vi "FGV_Kommunikation.vi"(8 "error in":errorcluster, 9 "termination char\n(0xA = '\\n' = LF)  2":u8=3 caption="Endzeichen\n(0xA = '\\n' = LF)" format="%.0x", 10 "Aktion":T1, 11 "VISA":refnum<visa-resource-name> caption="VISA-Ressourcenname") -> (0 "error out":errorcluster, 1 "Gase":cluster{string, i32}[][](array[cluster]), 3 "Device":string, 4 "Array 2":string[][][](array[string]), 5 "Array 3":string[][](array[string]))   [LabVIEW 2020, in "Linearisierung v2.lvlib" / "Gasteiler.lvlib" / "HovaCal.lvlib"]
uses:
  HovaCal.lvlib
  Aktion_FGV_Kom.ctl
  Aktion_txt.ctl
  Aktion_FGV_Betriebsdaten.ctl
  Betriebsdaten.ctl
  Vaporizer.ctl
  Dynamsiche_Werte.ctl
  <vilib>/Instr/_visa.llb/VISA Configure Serial Port (Instr).vi
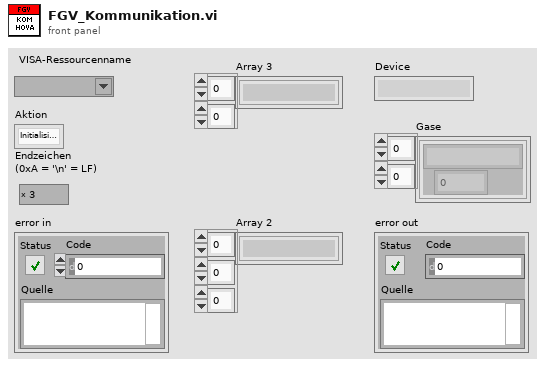
[diagram p1: front panel]
types:
  T1 = typedef "Linearisierung v2.lvlib/Gasteiler.lvlib/HovaCal.lvlib/Aktion_FGV_Kom.ctl" = enum16{"Initialisieren", "Betriebsparameter", "Gase", "Vaporizer", "Dynamische Werte", "Beenden", "Com ändern", "Gase init"}
  T2 = typedef "Linearisierung v2.lvlib/Gasteiler.lvlib/HovaCal.lvlib/Aktion_txt.ctl" = enum16{"ini", "lesen"}
  T3 = typedef "Linearisierung v2.lvlib/Gasteiler.lvlib/HovaCal.lvlib/Betriebsdaten.ctl" = cluster{"Gesamtdurchfluss":dbl, "Eingangskonzentration \nTrägergas":dbl, "Eingangskonzentration\nKomponente 1":dbl, "Eingangskonzentration \nKomponente 2":dbl, "Ausgangskonzentration \nKomponente 1 ":dbl, "Ausgangskonzentration\nKomponente 2":dbl, "l/min -> ml/min":bool, "N2 %->ppm":bool, "Komp1 ppm->%":bool, "Komp2ppm->%":bool, "Sollkomp1ppm->%":bool, "Sollkomp2ppm->%":bool}
  T4 = typedef "Linearisierung v2.lvlib/Gasteiler.lvlib/HovaCal.lvlib/Aktion_FGV_Betriebsdaten.ctl" = enum16{"Lesen", "Sollwerte schreiben", "Sollwerte lesen", "Gase schreiben", "Gase lesen", "Dynamische Werte", "GaseRef", "Gase aendern"}
  T5 = enum16{"Lesen", "Vaporizer lesen", "Vaporizer schreiben"}
  T6 = typedef "Linearisierung v2.lvlib/Gasteiler.lvlib/HovaCal.lvlib/Vaporizer.ctl" = cluster{"Pumpe Ein/Aus":dbl, "Wasser / Reagent":dbl, "Reagent dry / wet":dbl, "Reagent":dbl, "min. Temperatur\n160 °C":dbl, "Solltemperatur":dbl, "Wasserkonzentration\nSoll":dbl}
  T7 = typedef "Linearisierung v2.lvlib/Gasteiler.lvlib/HovaCal.lvlib/Dynamsiche_Werte.ctl" = cluster{"Durchfluss":dbl, "Drehzahl":dbl, "Wasserkonz.":dbl, "Ist - Temp":dbl, "Ist Konz 1":dbl, "Ist Konz 2":dbl}
  T8 = cluster{"Gesamtdurchfluss":bool, "Eingangskonzentration \nTrägergas":bool, "Eingangskonzentration\nKomponente 1":bool, "Eingangskonzentration \nKomponente 2":bool, "Ausgangskonzentration \nKomponente 1 ":bool, "Ausgangskonzentration\nKomponente 2":bool, "l/min -> ml/min":bool, "N2 %->ppm":bool, "Komp1 ppm->%":bool, "Komp2ppm->%":bool, "Sollkomp1ppm->%":bool, "Sollkomp2ppm->%":bool}
  T9 = typedef "Linearisierung v2.lvlib/Gasteiler.lvlib/HovaCal.lvlib/Gase.ctl" = cluster{"Trägergas":u16, "Komponente 1":u16, "Komponente 2":u16}
  T10 = cluster{"Pumpe Ein/Aus":bool, "Wasser / Reagent":bool, "Reagent dry / wet":bool, "Reagent":bool, "min. Temperatur\n160 °C":bool, "Solltemperatur":bool, "Wasserkonzentration\nSoll":bool}
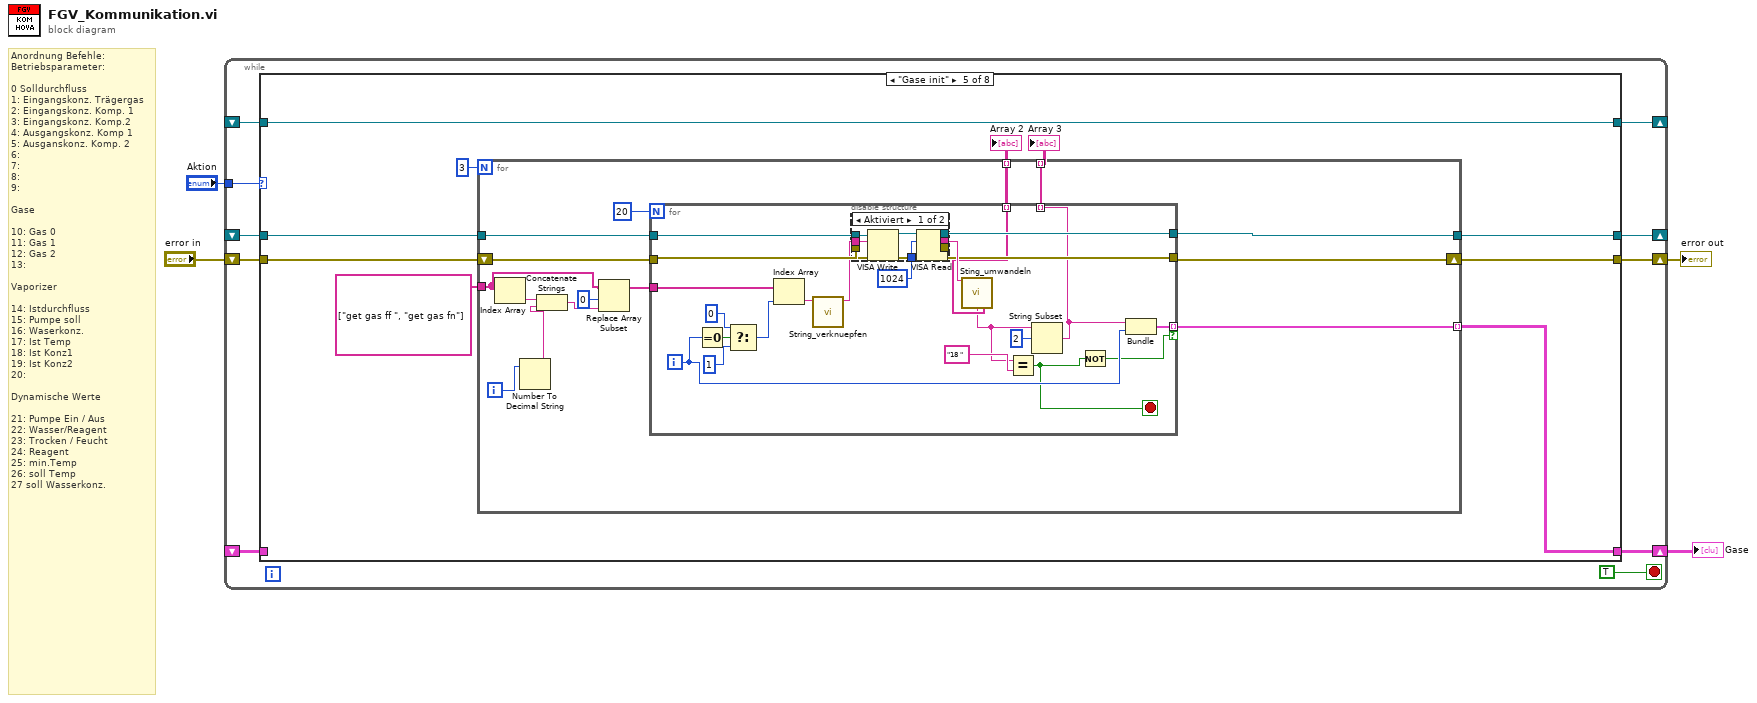
[diagram p0: block diagram]
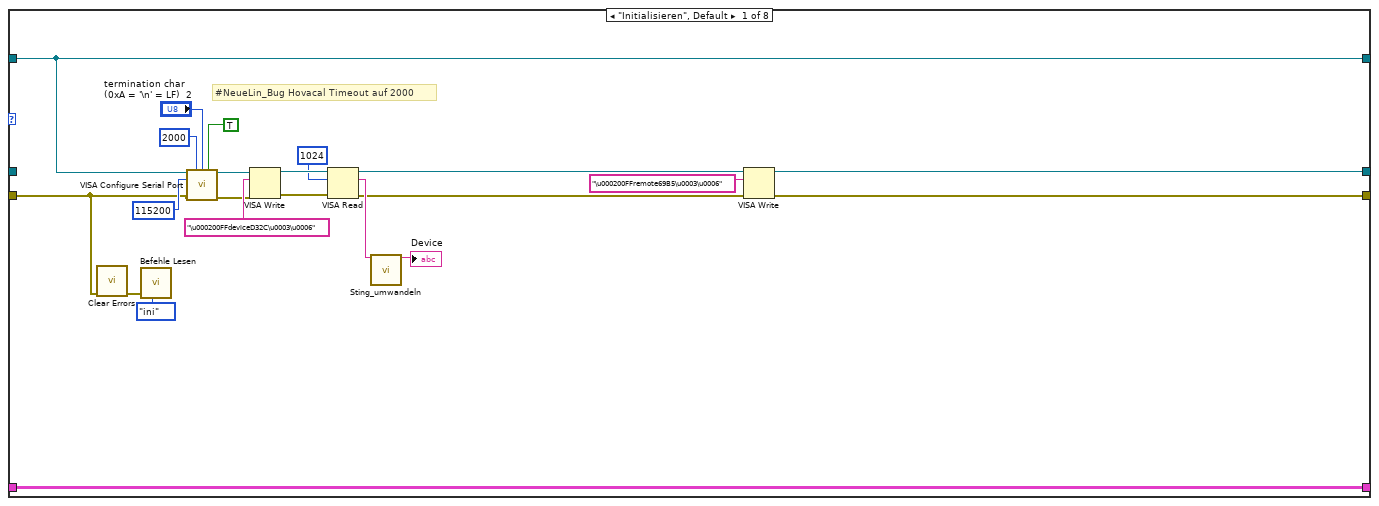
[diagram p2: hidden frame]
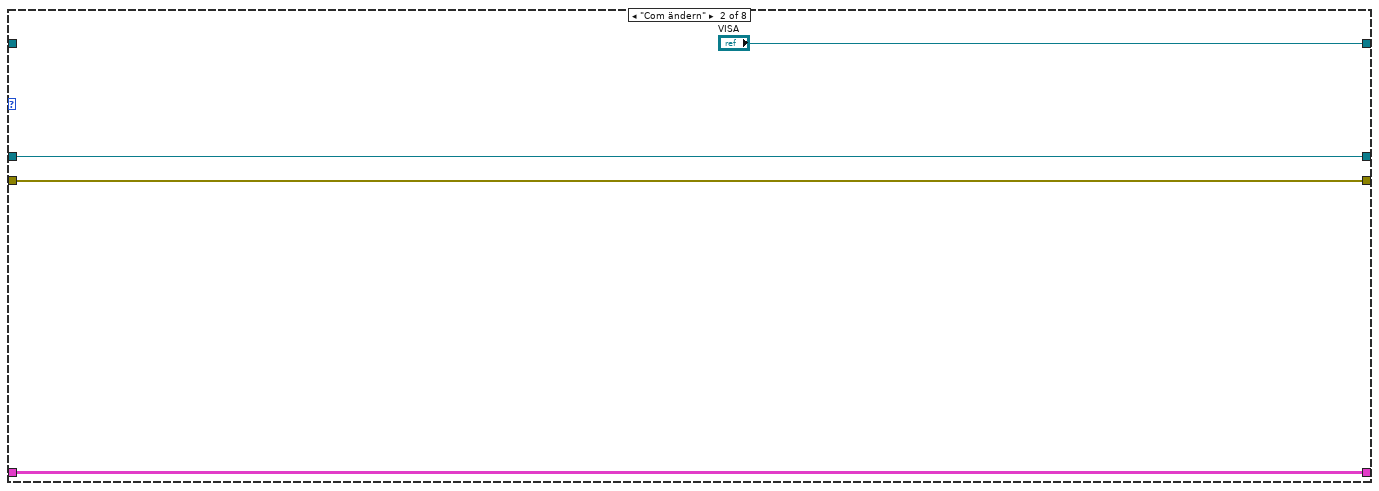
[diagram p3: hidden frame]
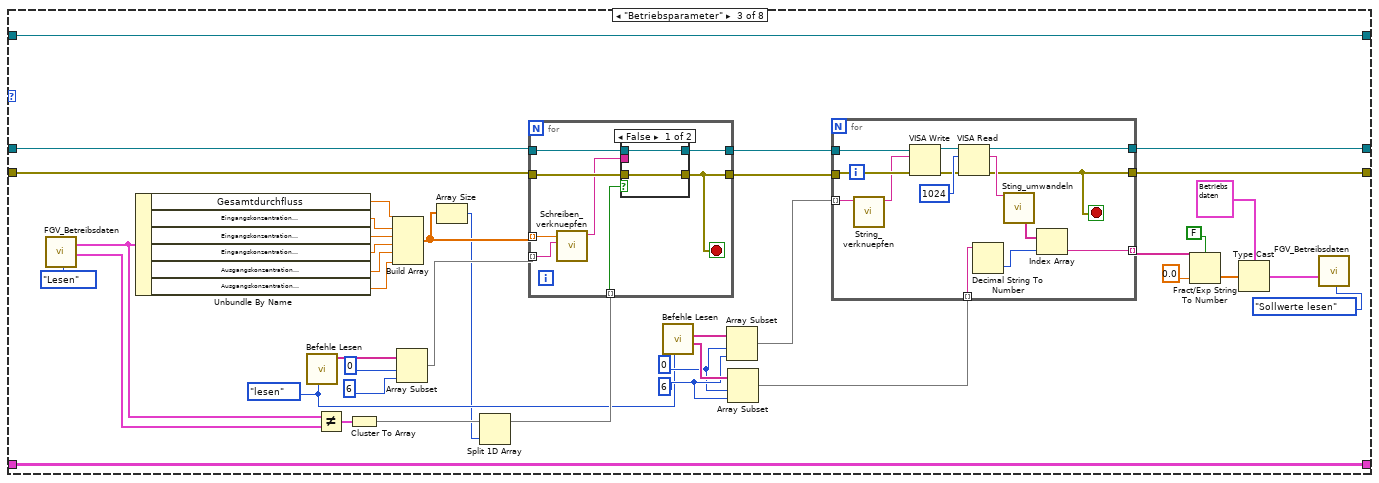
[diagram p4: hidden frame]
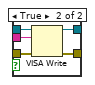
[diagram p5: hidden frame]
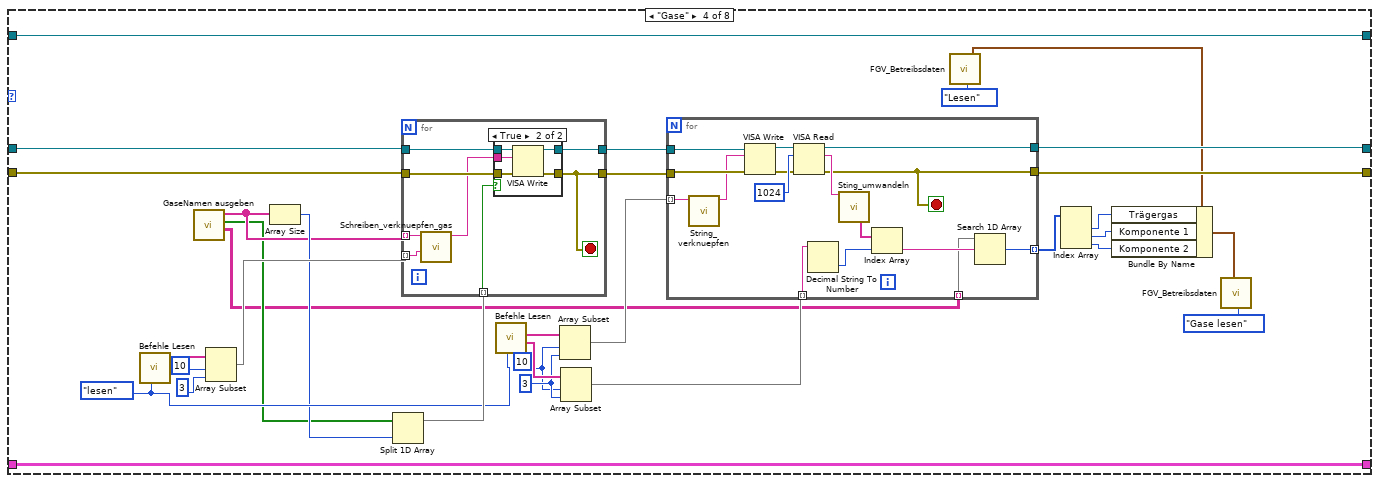
[diagram p6: hidden frame]
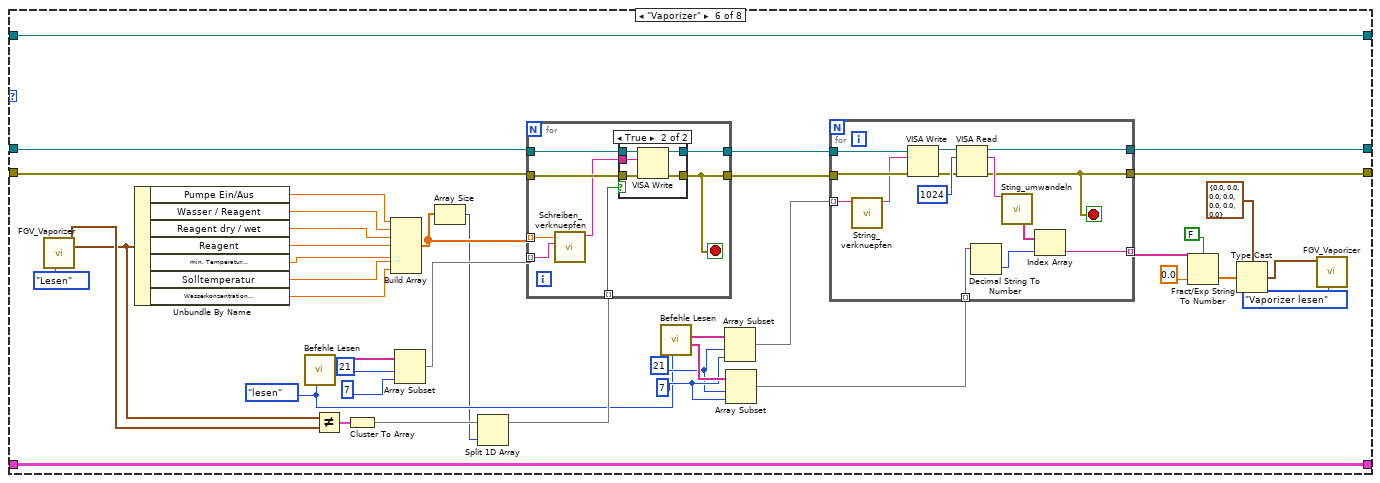
[diagram p9: hidden frame]
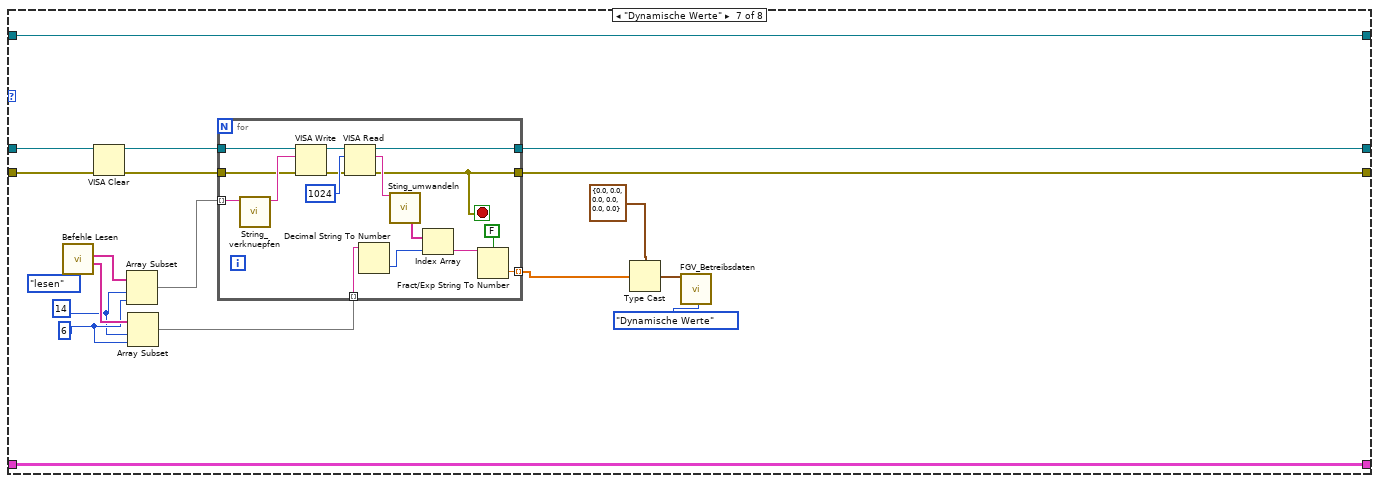
[diagram p11: hidden frame]
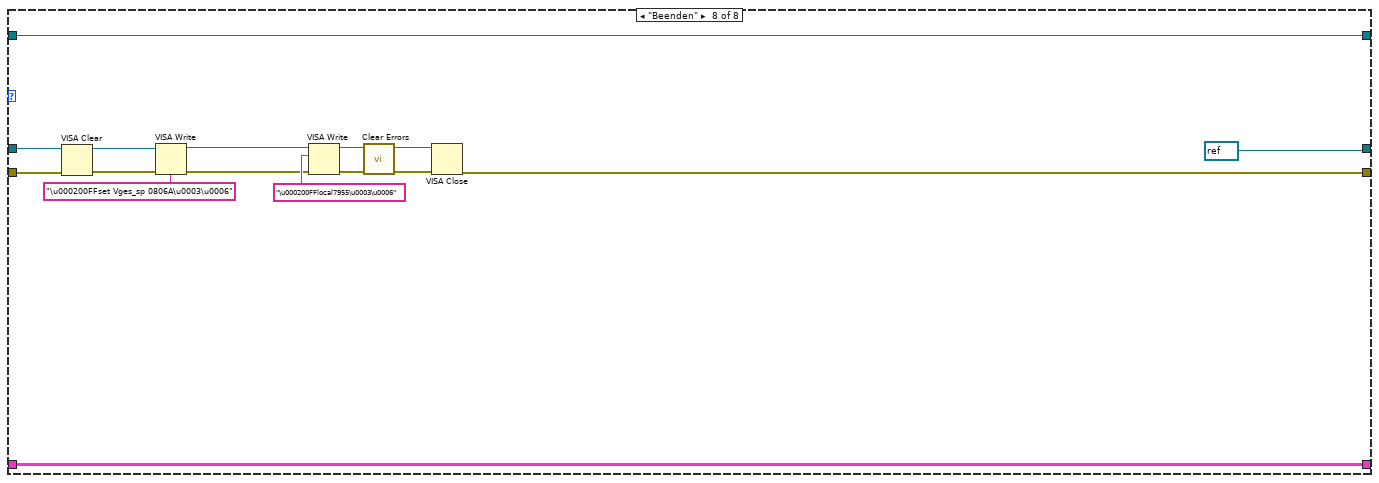
[diagram p12: hidden frame]
diagram:
  # "Anordnung Befehle:\nBetriebsparameter:\n\n0 Solldurchfluss\n1: Eingangskonz. Trägergas\n2: Eingangskonz. Komp. 1\n3: Eingangskonz. Komp.2\n4: Ausgangskonz. Komp 1\n5: Ausganskonz. Komp. 2\n6:\n7:\n8:\n9:\n\nGase\n\n10: Gas 0\n11: Gas 1\n12: Gas 2\n13:\n\nVaporizer\n\n14: Istdurchfluss\n15: Pumpe soll\n16: Waserkonz.\n17: Ist Temp\n18: Ist Konz1\n19: Ist Konz2\n20:\n\nDynamische Werte\n\n21: Pumpe Ein / Aus\n22: Wasser/Reagent\n23: Trocken / Feucht\n24: Reagent\n25: min.Temp\n26: soll Temp\n27 soll Wasserkonz."
  n1 = while {
    shift-right: [w13] -> _
    shift-left: _ -> [w11]
    shift-right: [w12] -> w4
    shift-left: "error in" -> [w10]
    tunnel: "Aktion" -> [w9]
    shift-right: [w8] -> _
    shift-left: _ -> [w7]
    shift-right: [w6] -> w1
    shift-left: _ -> [w5]
    stop <- TRUE stop-if-true
    n2 = case shown="\"Gase init\"" w9 {
      tunnel: [w24 w38 w69 w126 w180 w244 w308 refnum<visa-resource-name> refnum ("VISA resource name out")] -> w13
      tunnel: [w23 w40 w68 w125 w179 w243 w307 w336] -> w12
      tunnel: w11 -> [_ w38 w74 w128 w182 w246 w309 w340]
      tunnel: w10 -> [w15 w40 w75 w127 w181 w245 w304 w337]
      tunnel: [w18 "VISA" w44 w122 w178 w230 w302 w335] -> w8
      tunnel: w7 -> [w18 _ w44 w122 w178 w230 w302 w335]
      tunnel: [w17 w37 w41 w120 w175 w229 w300 w334] -> w6
      tunnel: w5 -> [w17 w37 w41 w120 _ w229 w300 w334]
      frame "Initialisieren", Default {
        # "#NeueLin_Bug Hovacal Timeout auf 2000"
        n3 = call <vilib>:"Clear Errors.vi"("error in (no error)"=w15) -> ("error out"=w16:errorcluster)  [unwired: 5 in, 1 out]
        n4 = call "Befehle Lesen.vi"("Enum"=Aktion_txt."ini", "error in"=w16) -> ()  [unwired: 6 in, 4 out]
        n5 = call-poly "VISA Configure Serial Port"("VISA resource name"=w18, "timeout (10sec)"=u32 2000, "termination char\n(0xA = '\\n' = LF)"="termination char\n(0xA = '\\n' = LF)  2", "Enable Termination\nChar (T)"=TRUE ("Enable Termination\nChar (T)"), "baud rate (9600)"=u32 115200, "error in (no error)"=w15) -> ("VISA resource name out"=w32:refnum<visa-resource-name>, "error out"=w31:errorcluster)  [unwired: 8 in]
        n6 = VISA Write(VISA resource name=w32, write buffer="\u000200FFdeviceD32C\u0003\u0006" ("Schreibpuffer"), error in (no error)=w31) -> (VISA resource name out=w35:refnum<visa-resource-name>, error out=w34:errorcluster)  [unwired: 1 out]
        n7 = VISA Read(VISA resource name=w35, byte count=u32 1024 ("Byte-Anzahl"), error in (no error)=w34) -> (VISA resource name out=w22:refnum<visa-resource-name>, read buffer=w30:string, error out=w21:errorcluster)  [unwired: 1 out]
        n8 = call "Sting_umwandeln.vi"("Lesepuffer"=w30) -> ("Device"=→"Device":string)  [unwired: 8 in, 6 out]
        n9 = VISA Write(VISA resource name=w22, write buffer="\u000200FFremote69B5\u0003\u0006" ("Schreibpuffer"), error in (no error)=w21) -> (VISA resource name out=w24:refnum<visa-resource-name>, error out=w23:errorcluster)  [unwired: 1 out]
      }
      frame "Com ändern" {
      }
      frame "Betriebsparameter" {
        w49 = Aktion_txt."lesen" ("Enum")
        w65 = 6 ("Index")
        w64 = 0 ("Index")
        n10 = call "FGV_Betreibsdaten.vi"("Enum"=Aktion_FGV_Betriebsdaten."Lesen") -> ("Sollwerte schreiben"=w45:T3, "Sollwerte lesen"=w78:T3)  [unwired: 11 in, 6 out]
        n11 = Unbundle By Name(w45) -> ("Gesamtdurchfluss"=w57:dbl, "Eingangskonzentration \nTrägergas"=w56:dbl, "Eingangskonzentration\nKomponente 1"=w55:dbl, "Eingangskonzentration \nKomponente 2"=w54:dbl, "Ausgangskonzentration \nKomponente 1"=w53:dbl, "Ausgangskonzentration\nKomponente 2"=w52:dbl)
        n12 = call "Befehle Lesen.vi"("Enum"=w49) -> ("Schreibbefehl"=w77:string[])  [unwired: 7 in, 3 out]
        n13 = Not Equal?(x=w45, y=w78) -> (x != y?=w51:T8)
        n14 = Cluster To Array(cluster=w51) -> (array=w50:bool[])
        n15 = Build Array(w57, w56, w55, w54, w53, w52) -> (w72:dbl[])
        n16 = Array Subset(array=w77, index=0 ("Index"), length=6 ("Länge")) -> (w73:string[])
        n17 = Array Size(array=w72) -> (size(s)=w48:i32)
        n18 = Split 1D Array(array=w50, index=w48) -> (first subarray=w76:bool[])  [unwired: 1 out]
        n19 = for {
          tunnel: w74 -> [w101]
          tunnel: w75 -> [w100]
          tunnel: [w102] -> w71
          tunnel: [w99] -> w70
          tunnel: w76 -> [w98] mode=indexing
          tunnel: w73 -> [w96] mode=indexing
          tunnel: w72 -> [w97] mode=indexing
          stop <- w99 stop-if-true
          n20 = call "Schreiben_verknuepfen.vi"("Order"=w96, "Zahl"=w97) -> ("Verknüpfter String"=w95:string)  [unwired: 8 in, 1 out]
          n21 = case shown="False" w98 {
            tunnel: [w104 w109] -> w102
            tunnel: w101 -> [w104 w108]
            tunnel: w100 -> [w103 w107]
            tunnel: w95 -> [_ w106]
            tunnel: [w103 w105] -> w99
            frame False {
            }
            frame True {
              n22 = VISA Write(VISA resource name=w108, write buffer=w106, error in (no error)=w107) -> (VISA resource name out=w109:refnum<visa-resource-name>, error out=w105:errorcluster)  [unwired: 1 out]
            }
          }
        }
        n23 = call "Befehle Lesen.vi"("Enum"=w49) -> ("Ausgang für Lesen"=w66:string[], "Lesebefehl"=w67:string[])  [unwired: 7 in, 2 out]
        n24 = Array Subset(array=w67, index=w64, length=w65) -> (w63:string[])
        n25 = Array Subset(array=w66, index=w64, length=w65) -> (w62:string[])
        n26 = for {
          tunnel: w71 -> [w94]
          tunnel: w70 -> [w93]
          tunnel: w63 -> [w84] mode=indexing
          tunnel: [w89] -> w69
          tunnel: [w85] -> w68
          tunnel: w62 -> [w87] mode=indexing
          tunnel: [w86] -> w59 mode=indexing
          stop <- w85 stop-if-true
          n27 = call "String_verknuepfen.vi"("Order"=w84) -> ("Verknüpfter String"=w83:string)  [unwired: 9 in, 1 out]
          n28 = VISA Write(VISA resource name=w94, write buffer=w83, error in (no error)=w93) -> (VISA resource name out=w91:refnum<visa-resource-name>, error out=w90:errorcluster)  [unwired: 1 out]
          n29 = VISA Read(VISA resource name=w91, byte count=u32 1024 ("Byte-Anzahl"), error in (no error)=w90) -> (VISA resource name out=w89:refnum<visa-resource-name>, read buffer=w88:string, error out=w85:errorcluster)  [unwired: 1 out]
          n30 = Decimal String To Number(string=w87) -> (number=w81:i32)  [unwired: 2 in, 1 out]
          n31 = call "Sting_umwandeln.vi"("Lesepuffer"=w88) -> ("Array"=w82:string[])  [unwired: 8 in, 6 out]
          n32 = Index Array(array=w82, index=w81) -> (element=w86:string)
        }
        n33 = Fract/Exp String To Number(use system decimal point (T)=FALSE ("Systemdezimalzeichen verwenden (T)"), string=w59, default (0 dbl)=0.0 ("Standard (0 I32)")) -> (number=w60:dbl[])  [unwired: 1 in, 1 out]
        n34 = Type Cast(type=T3 {"Gesamtdurchfluss"=0.0, "Eingangskonzentration \nTrägergas"=0.0, "Eingangskonzentration\nKomponente 1"=0.0, "Eingangskonzentration \nKomponente 2"=0.0, "Ausgangskonzentration \nKomponente 1 "=0.0, "Ausgangskonzentration\nKomponente 2"=0.0, "l/min -> ml/min"=FALSE, "N2 %->ppm"=FALSE, "Komp1 ppm->%"=FALSE, "Komp2ppm->%"=FALSE, "Sollkomp1ppm->%"=FALSE, "Sollkomp2ppm->%"=FALSE} ("Daten"), x=w60) -> (*(type *) &x=w46:T3)
        n35 = call "FGV_Betreibsdaten.vi"("Sollwerte lesen"=w46, "Enum"=Aktion_FGV_Betriebsdaten."Sollwerte lesen") -> ()  [unwired: 10 in, 8 out]
      }
      frame "Gase" {
        w124 = Aktion_txt."lesen" ("Enum")
        w132 = 3 ("Index")
        w131 = 10 ("Index")
        n36 = call "Befehle Lesen.vi"("Enum"=w124) -> ("Schreibbefehl"=w139:string[])  [unwired: 7 in, 3 out]
        n37 = call "GaseNamen ausgeben.vi"() -> ("Komplettes Enum in String"=w116:string[][], "Vergleich"=w118:bool[], "GaseArray"=w119:string[])  [unwired: 8 in, 1 out]
        n38 = Array Subset(array=w139, index=10 ("Index"), length=3 ("Länge")) -> (w137:string[])
        n39 = Array Size(array=w119) -> (size(s)=w123:i32)
        n40 = Split 1D Array(array=w118, index=w123) -> (first subarray=w138:bool[])  [unwired: 1 out]
        n41 = for {
          tunnel: w128 -> [w164]
          tunnel: w127 -> [w163]
          tunnel: [w165] -> w136
          tunnel: [w162] -> w135
          tunnel: w138 -> [w161] mode=indexing
          tunnel: w137 -> [w159] mode=indexing
          tunnel: w119 -> [w160] mode=indexing
          stop <- w162 stop-if-true
          n42 = call "Schreiben_verknuepfen_gas.vi"("Order"=w159, "gas"=w160) -> ("Verknüpfter String"=w158:string)  [unwired: 8 in, 1 out]
          n43 = case shown="True" w161 {
            tunnel: [w167 w172] -> w165
            tunnel: w164 -> [w167 w171]
            tunnel: w163 -> [w166 w170]
            tunnel: w158 -> [_ w169]
            tunnel: [w166 w168] -> w162
            frame False {
            }
            frame True {
              n44 = VISA Write(VISA resource name=w171, write buffer=w169, error in (no error)=w170) -> (VISA resource name out=w172:refnum<visa-resource-name>, error out=w168:errorcluster)  [unwired: 1 out]
            }
          }
        }
        n45 = call "Befehle Lesen.vi"("Enum"=w124) -> ("Ausgang für Lesen"=w133:string[], "Lesebefehl"=w134:string[])  [unwired: 7 in, 2 out]
        n46 = Array Subset(array=w134, index=w131, length=w132) -> (w130:string[])
        n47 = Array Subset(array=w133, index=w131, length=w132) -> (w129:string[])
        n48 = for {
          tunnel: w136 -> [w157]
          tunnel: w135 -> [w156]
          tunnel: w130 -> [w148] mode=indexing
          tunnel: [w152] -> w126
          tunnel: [w149] -> w125
          tunnel: w129 -> [w150] mode=indexing
          tunnel: w116 -> [w143] mode=indexing
          tunnel: [w142] -> w113 mode=indexing
          stop <- w149 stop-if-true
          n49 = call "String_verknuepfen.vi"("Order"=w148) -> ("Verknüpfter String"=w147:string)  [unwired: 9 in, 1 out]
          n50 = VISA Write(VISA resource name=w157, write buffer=w147, error in (no error)=w156) -> (VISA resource name out=w154:refnum<visa-resource-name>, error out=w153:errorcluster)  [unwired: 1 out]
          n51 = VISA Read(VISA resource name=w154, byte count=u32 1024 ("Byte-Anzahl"), error in (no error)=w153) -> (VISA resource name out=w152:refnum<visa-resource-name>, read buffer=w151:string, error out=w149:errorcluster)  [unwired: 1 out]
          n52 = Decimal String To Number(string=w150) -> (number=w145:i32)  [unwired: 2 in, 1 out]
          n53 = call "Sting_umwandeln.vi"("Lesepuffer"=w151) -> ("Array"=w146:string[])  [unwired: 8 in, 6 out]
          n54 = Index Array(array=w146, index=w145) -> (element=w144:string)
          n55 = Search 1D Array(1D array=w143, element=w144) -> (index of element=w142:i32)  [unwired: 1 in]
        }
        n56 = call "FGV_Betreibsdaten.vi"("Enum"=Aktion_FGV_Betriebsdaten."Lesen") -> ("Gase lesen"=w115:T9)  [unwired: 11 in, 7 out]
        n57 = Index Array(array=w113) -> (element #1=w112:i32, element #2=w111:i32, element #3=w110:i32)  [unwired: 3 in]
        n58 = Bundle By Name(cluster=w115, "Trägergas"=w112, "Komponente 1"=w111, "Komponente 2"=w110) -> (w114:T9)
        n59 = call "FGV_Betreibsdaten.vi"("Gase lesen"=w114, "Enum"=Aktion_FGV_Betriebsdaten."Gase lesen") -> ()  [unwired: 10 in, 8 out]
      }
      frame "Gase init" {
        n60 = for {
          N: 3 -> [_]
          tunnel: w182 -> [w197]
          tunnel: [w195] -> w180
          tunnel: string[] ["get gas ff ", "get gas fn"] -> [w189]
          shift-right: [w194] -> w179
          shift-left: w181 -> [w196]
          tunnel: [w183] -> w175 mode=indexing
          tunnel: [w185] -> w174 mode=indexing
          tunnel: [w184] -> w173 mode=indexing
          i -> [w186]
          n61 = Index Array(array=w189) -> (element=w193:string)  [unwired: 1 in]
          n62 = Number To Decimal String(number=w186) -> (decimal integer string=w192:string)  [unwired: 1 in]
          n63 = Concatenate Strings(w193, w192) -> (w190:string)
          n64 = Replace Array Subset(array=w189, new element=w190, index=0 ("Index")) -> (w191:string[])
          n65 = for {
            N: 20 -> [_]
            tunnel: w197 -> [w219]
            tunnel: w196 -> [w218]
            tunnel: [w216] -> w195
            tunnel: [w214] -> w194
            tunnel: w191 -> [w212]
            tunnel: [w205] -> w183 mode=indexing if=w198
            tunnel: [w204] -> w185 mode=indexing
            tunnel: [w202] -> w184 mode=indexing
            i -> [w206]
            stop <- w199 stop-if-true
            n66 = Equal To 0?(x=w206) -> (x = 0?=w211:bool)
            n67 = Select(t=0 ("Index"), s=w211, f=1 ("Index")) -> (s? t:f=w208:i32)
            n68 = Index Array(array=w212, index=w208) -> (element=w207:string)
            n69 = call "String_verknuepfen.vi"("Order"=w207) -> ("Verknüpfter String"=w213:string)  [unwired: 9 in, 1 out]
            n70 = disable-structure shown="Aktiviert" {
              disable-tunnel: w219 -> [w228 _]
              disable-tunnel: w218 -> [w227 _]
              disable-tunnel: u32 1024 ("Byte-Anzahl") -> [w226 _]
              disable-tunnel: [w223 _] -> w216
              disable-tunnel: [w222 _] -> w215
              disable-tunnel: [w221 _] -> w214
              disable-tunnel: w213 -> [w220 _]
              frame Enabled {
                n71 = VISA Write(VISA resource name=w228, write buffer=w220, error in (no error)=w227) -> (VISA resource name out=w225:refnum<visa-resource-name>, error out=w224:errorcluster)  [unwired: 1 out]
                n72 = VISA Read(VISA resource name=w225, byte count=w226, error in (no error)=w224) -> (VISA resource name out=w223:refnum<visa-resource-name>, read buffer=w222:string, error out=w221:errorcluster)  [unwired: 1 out]
              }
              frame Disabled {
              }
            }
            n73 = call "Sting_umwandeln.vi"("Lesepuffer"=w215) -> ("Gase"=w200:string, "Array"=w204:string[])  [unwired: 8 in, 5 out]
            n74 = Equal?(x=w200, y="18 ") -> (x = y?=w199:bool)
            n75 = String Subset(string=w200, offset (0)=2 ("Offset (0)")) -> (substring=w202:string)  [unwired: 1 in]
            n76 = Not(x=w199) -> (.not. x?=w198:bool)
            n77 = Bundle("Gase"=w202, w206) -> (w205:cluster{"Gase":string, i32})  [unwired: 1 in]
          }
        }
        "Array 2" <- w174
        "Array 3" <- w173
      }
      frame "Vaporizer" {
        w249 = Aktion_txt."lesen" ("Enum")
        w259 = 7 ("Index")
        w258 = 21 ("Index")
        n78 = call "FGV_Vaporizer.vi"("Enum"=T5."Lesen") -> ("Vaporizer_schreiben"=w240:T6, "Vaporizer_lesen"=w242:T6)  [unwired: 7 in, 2 out]
        n79 = Unbundle By Name(w240) -> ("Pumpe Ein/Aus"=w239:dbl, "Wasser / Reagent"=w238:dbl, "Reagent dry / wet"=w237:dbl, "Reagent"=w231:dbl, "min. Temperatur\n160 °C"=w236:dbl, "Solltemperatur"=w235:dbl, "Wasserkonzentration\nSoll"=w234:dbl)
        n80 = call "Befehle Lesen.vi"("Enum"=w249) -> ("Schreibbefehl"=w267:string[])  [unwired: 7 in, 3 out]
        n81 = Not Equal?(x=w240, y=w242) -> (x != y?=w251:T10)
        n82 = Cluster To Array(cluster=w251) -> (array=w250:bool[])
        n83 = Build Array(w239, w238, w237, w231, w236, w235, w234) -> (w264:dbl[])
        n84 = Array Subset(array=w267, index=21 ("Index"), length=7 ("Länge")) -> (w265:string[])
        n85 = Array Size(array=w264) -> (size(s)=w248:i32)
        n86 = Split 1D Array(array=w250, index=w248) -> (first subarray=w266:bool[])  [unwired: 1 out]
        n87 = for {
          tunnel: w246 -> [w290]
          tunnel: w245 -> [w289]
          tunnel: [w291] -> w263
          tunnel: [w288] -> w262
          tunnel: w266 -> [w287] mode=indexing
          tunnel: w265 -> [w285] mode=indexing
          tunnel: w264 -> [w286] mode=indexing
          stop <- w288 stop-if-true
          n88 = call "Schreiben_verknuepfen.vi"("Order"=w285, "Zahl"=w286) -> ("Verknüpfter String"=w284:string)  [unwired: 8 in, 1 out]
          n89 = case shown="True" w287 {
            tunnel: [w293 w298] -> w291
            tunnel: w290 -> [w293 w297]
            tunnel: w289 -> [w292 w296]
            tunnel: w284 -> [_ w295]
            tunnel: [w292 w294] -> w288
            frame False {
            }
            frame True {
              n90 = VISA Write(VISA resource name=w297, write buffer=w295, error in (no error)=w296) -> (VISA resource name out=w298:refnum<visa-resource-name>, error out=w294:errorcluster)  [unwired: 1 out]
            }
          }
        }
        n91 = call "Befehle Lesen.vi"("Enum"=w249) -> ("Ausgang für Lesen"=w260:string[], "Lesebefehl"=w261:string[])  [unwired: 7 in, 2 out]
        n92 = Array Subset(array=w261, index=w258, length=w259) -> (w257:string[])
        n93 = Array Subset(array=w260, index=w258, length=w259) -> (w256:string[])
        n94 = for {
          tunnel: w263 -> [w283]
          tunnel: w262 -> [w282]
          tunnel: w257 -> [w273] mode=indexing
          tunnel: [w278] -> w244
          tunnel: [w274] -> w243
          tunnel: w256 -> [w276] mode=indexing
          tunnel: [w275] -> w253 mode=indexing
          stop <- w274 stop-if-true
          n95 = call "String_verknuepfen.vi"("Order"=w273) -> ("Verknüpfter String"=w272:string)  [unwired: 9 in, 1 out]
          n96 = VISA Write(VISA resource name=w283, write buffer=w272, error in (no error)=w282) -> (VISA resource name out=w280:refnum<visa-resource-name>, error out=w279:errorcluster)  [unwired: 1 out]
          n97 = VISA Read(VISA resource name=w280, byte count=u32 1024 ("Byte-Anzahl"), error in (no error)=w279) -> (VISA resource name out=w278:refnum<visa-resource-name>, read buffer=w277:string, error out=w274:errorcluster)  [unwired: 1 out]
          n98 = Decimal String To Number(string=w276) -> (number=w270:i32)  [unwired: 2 in, 1 out]
          n99 = call "Sting_umwandeln.vi"("Lesepuffer"=w277) -> ("Array"=w271:string[])  [unwired: 8 in, 6 out]
          n100 = Index Array(array=w271, index=w270) -> (element=w275:string)
        }
        n101 = Fract/Exp String To Number(use system decimal point (T)=FALSE ("Systemdezimalzeichen verwenden (T)"), string=w253, default (0 dbl)=0.0 ("Standard (0 I32)")) -> (number=w254:dbl[])  [unwired: 1 in, 1 out]
        n102 = Type Cast(type=T6 {"Pumpe Ein/Aus"=0.0, "Wasser / Reagent"=0.0, "Reagent dry / wet"=0.0, "Reagent"=0.0, "min. Temperatur\n160 °C"=0.0, "Solltemperatur"=0.0, "Wasserkonzentration\nSoll"=0.0} ("Vaporizer"), x=w254) -> (*(type *) &x=w232:T6)
        n103 = call "FGV_Vaporizer.vi"("Enum"=T5."Vaporizer lesen", "Vaporizer lesen"=w232) -> ()  [unwired: 6 in, 4 out]
      }
      frame "Dynamische Werte" {
        w315 = 6 ("Index")
        w314 = 14 ("Index")
        n104 = call "Befehle Lesen.vi"("Enum"=Aktion_txt."lesen") -> ("Ausgang für Lesen"=w316:string[], "Lesebefehl"=w317:string[])  [unwired: 7 in, 2 out]
        n105 = VISA Clear(VISA resource name=w309, error in (no error)=w304) -> (VISA resource name out=w305:refnum<visa-resource-name>, error out=w303:errorcluster)
        n106 = Array Subset(array=w317, index=w314, length=w315) -> (w313:string[])
        n107 = Array Subset(array=w316, index=w314, length=w315) -> (w312:string[])
        n108 = for {
          tunnel: w313 -> [w326] mode=indexing
          tunnel: [w330] -> w308
          tunnel: [w327] -> w307
          tunnel: w312 -> [w328] mode=indexing
          tunnel: w305 -> [w322]
          tunnel: w303 -> [w321]
          tunnel: [w319] -> w299 mode=indexing
          stop <- w327 stop-if-true
          n109 = call "String_verknuepfen.vi"("Order"=w326) -> ("Verknüpfter String"=w325:string)  [unwired: 9 in, 1 out]
          n110 = VISA Write(VISA resource name=w322, write buffer=w325, error in (no error)=w321) -> (VISA resource name out=w332:refnum<visa-resource-name>, error out=w331:errorcluster)  [unwired: 1 out]
          n111 = VISA Read(VISA resource name=w332, byte count=u32 1024 ("Byte-Anzahl"), error in (no error)=w331) -> (VISA resource name out=w330:refnum<visa-resource-name>, read buffer=w329:string, error out=w327:errorcluster)  [unwired: 1 out]
          n112 = Decimal String To Number(string=w328) -> (number=w323:i32)  [unwired: 2 in, 1 out]
          n113 = call "Sting_umwandeln.vi"("Lesepuffer"=w329) -> ("Array"=w324:string[])  [unwired: 8 in, 6 out]
          n114 = Index Array(array=w324, index=w323) -> (element=w320:string)
          n115 = Fract/Exp String To Number(use system decimal point (T)=FALSE ("Systemdezimalzeichen verwenden (T)"), string=w320) -> (number=w319:dbl)  [unwired: 2 in, 1 out]
        }
        n116 = Type Cast(type=T7 {"Durchfluss"=0.0, "Drehzahl"=0.0, "Wasserkonz."=0.0, "Ist - Temp"=0.0, "Ist Konz 1"=0.0, "Ist Konz 2"=0.0} ("Dynamische Werte"), x=w299) -> (*(type *) &x=w311:T7)
        n117 = call "FGV_Betreibsdaten.vi"("Dynamische Werte"=w311, "Enum"=Aktion_FGV_Betriebsdaten."Dynamische Werte" ("Aktion")) -> ()  [unwired: 10 in, 8 out]
      }
      frame "Beenden" {
        n118 = VISA Clear(VISA resource name=w340, error in (no error)=w337) -> (VISA resource name out=w339:refnum<visa-resource-name>, error out=w338:errorcluster)
        n119 = VISA Write(VISA resource name=w339, write buffer="\u000200FFset Vges_sp 0806A\u0003\u0006" ("Schreibpuffer"), error in (no error)=w338) -> (VISA resource name out=w342:refnum<visa-resource-name>, error out=w344:errorcluster)  [unwired: 1 out]
        n120 = VISA Write(VISA resource name=w342, write buffer="\u000200FFlocal7955\u0003\u0006" ("Schreibpuffer"), error in (no error)=w344) -> (VISA resource name out=w343:refnum<visa-resource-name>, error out=w346:errorcluster)  [unwired: 1 out]
        n121 = call <vilib>:"Clear Errors.vi"("error in (no error)"=w346) -> ("error out"=w347:errorcluster)  [unwired: 5 in, 1 out]
        n122 = VISA Close(VISA resource name=w343, error in (no error)=w347) -> (error out=w336:errorcluster)
      }
    }
  }
  "error out" <- w4
  "Gase" <- w1
